vi "PDF-Create Catalog.vi"(0 "PDF Path":path=path "C:/Users/hancock/Desktop/test.pdf", 5 "VI":refnum<vi>, 7 "Rows":i32=1, 9 "Cols":i32=1, 11 "error in (no error)":errorcluster) -> (4 "catalog":T1, 15 "error out":errorcluster)   [LabVIEW 2020]
uses:
  <vilib>/Exaprom PDF/Controls/Page Controls/Page size.ctl
  <vilib>/Exaprom PDF/Controls/Page Controls/Page Orientation.ctl
  <vilib>/Exaprom PDF/Controls/Page Controls/Page Layout Custom.ctl
  <vilib>/Exaprom PDF/Controls/Page Controls/Page margins.ctl
  <vilib>/Exaprom PDF/Controls/Page Controls/Page setup.ctl
  <userlib>/Exaprom PDF/Controls/Initialization Controls/At the opening.ctl
  <vilib>/Exaprom PDF/LV Class/PDF Report Class/PDF Report Class.lvclass
  PDF-Catalog.ctl
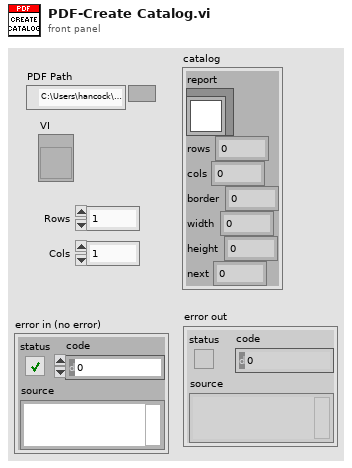
[diagram p1: front panel]
types:
  T1 = typedef "PDF-Catalog.ctl" = cluster{"report":refnum<class "PDF Report Class.lvclass">, "rows":i32, "cols":i32, "border":dbl, "width":dbl, "height":dbl, "next":i32}
  T2 = typedef "At the opening.ctl" = cluster{"Page":u16, "Show Bookmarks":bool}
  T3 = typedef "Page setup.ctl" = cluster{"Page Size":T4, "Orientation":T5, "Custom Size":T6, "Margins":T7}
  T4 = typedef "Page size.ctl" = i32
  T5 = typedef "Page Orientation.ctl" = enum16{"Portrait", "Landscape"}
  T6 = typedef "Page Layout Custom.ctl" = cluster{"Width":sgl, "Height":sgl}
  T7 = typedef "Page margins.ctl" = cluster{"Left":sgl, "Right":sgl, "Top":sgl, "Bottom":sgl}
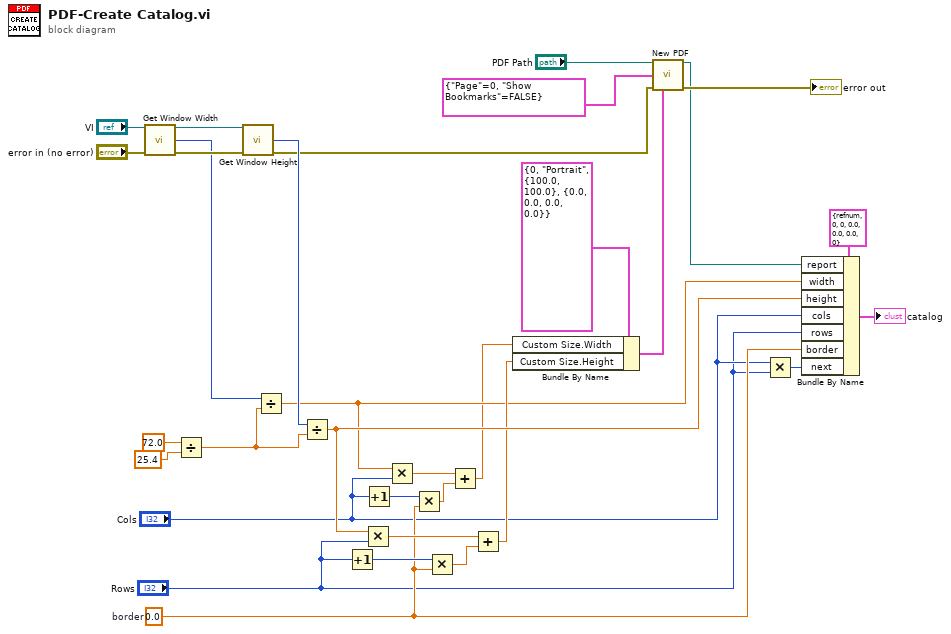
[diagram p0: block diagram]
diagram:
  w4 = 0.0  # border
  n1 = call "Get Window Width.vi"("VI in"="VI", "error in (no error)"="error in (no error)") -> ("VI out"=w28:refnum<vi>, "Width"=w24:i16, "error out"=w29:errorcluster)  [unwired: 11 in]
  n2 = Divide(x=72.0, y=25.4) -> (x/y=w23:dbl)
  n3 = call "Get Window Height.vi"("VI in"=w28, "error in (no error)"=w29) -> ("Height"=w25:i16, "error out"=w20:errorcluster)  [unwired: 11 in, 1 out]
  n4 = Divide(x=w24, y=w23) -> (x/y=w6:dbl)
  n5 = Divide(x=w25, y=w23) -> (x/y=w15:dbl)
  n6 = Increment(x="Rows") -> (x+1=w14:i32)
  n7 = Multiply(x=w15, y="Rows") -> (x*y=w12:dbl)
  n8 = Increment(x="Cols") -> (x+1=w9:i32)
  n9 = Multiply(x=w6, y="Cols") -> (x*y=w7:dbl)
  n10 = Multiply(x=w9, y=w4) -> (x*y=w8:dbl)
  n11 = Multiply(x=w14, y=w4) -> (x*y=w13:dbl)
  n12 = Add(x=w7, y=w8) -> (x+y=w5:dbl)
  n13 = Add(x=w12, y=w13) -> (x+y=w11:dbl)
  n14 = Bundle By Name(cluster=T3 {"Page Size"=0, "Orientation"=enum."Portrait", "Custom Size"={"Width"=100.0, "Height"=100.0}, "Margins"={"Left"=0.0, "Right"=0.0, "Top"=0.0, "Bottom"=0.0}} ("Page Setup"), "Custom Size.Width"=w5, "Custom Size.Height"=w11) -> (w22:T3)
  n15 = call <vilib>:"New PDF.vi"("PDF Path"="PDF Path", "At the opening"=T2 {"Page"=0, "Show Bookmarks"=FALSE}, "error in (no error)"=w20, "Page Setup"=w22) -> ("PDF Report"=w16:refnum<class "PDF Report Class.lvclass">, "error out"=→"error out":errorcluster)  [unwired: 10 in]
  n16 = Multiply(x="Cols", y="Rows") -> (x*y=w1:i32)
  n17 = Bundle By Name(cluster=T1 {"report"=refnum, "rows"=0, "cols"=0, "border"=0.0, "width"=0.0, "height"=0.0, "next"=0} ("catalog"), "report"=w16, "width"=w6, "height"=w15, "cols"="Cols", "rows"="Rows", "border"=w4, "next"=w1) -> (→"catalog":T1)
